vi "readEndOfFrame.vi"(8 "error in (no error)":errorcluster, 11 "ModbusBuffer in":refnum<class "ModbusBufferBuilder.lvclass">) -> (0 "error out":errorcluster, 3 "ModbusBuffer out":refnum<class "ModbusBufferBuilder.lvclass">)   [LabVIEW 2016, in "ModbusBufferBuilder.lvclass"]
uses:
  ModbusBufferBuilder.lvclass
  ModbusBufferBuilder.lvclass/ModbusBufferBuilder.ctl
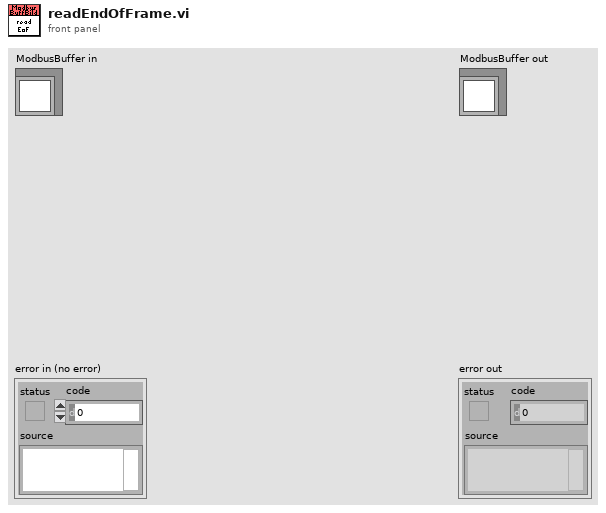
[diagram p1: front panel]
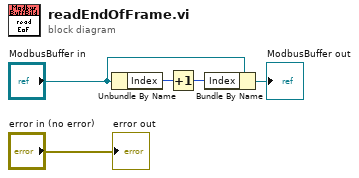
[diagram p0: block diagram]
diagram:
  n1 = Unbundle By Name("ModbusBuffer in") -> ("Index"=w3:i32)
  n2 = Increment(x=w3) -> (x+1=w2:i32)
  n3 = Bundle By Name(cluster="ModbusBuffer in", "Index"=w2) -> (→"ModbusBuffer out":refnum<class "ModbusBufferBuilder.lvclass">)
  "error out" <- "error in (no error)"
